vi "1_1_FFT and components.vi"() -> ()   [LabVIEW 2009]
doc: "This program calculates the magnitude spectrum, phase spectrum, real and imaginary spectrum of a sequence defined by the \"SIGNAL\" option menu."
uses:
  <vilib>/measure/matone.llb/Extract Single Tone Information 1 Chan.vi
  <vilib>/Analysis/2dsp.llb/Real FFT.vi
  <vilib>/Analysis/4window.llb/Hanning Window (DBL).vi
  <vilib>/Analysis/4window.llb/Hamming Window (DBL).vi
  <vilib>/Analysis/4window.llb/Triangle Window (DBL).vi
  <vilib>/Analysis/4window.llb/Kaiser-Bessel Window (DBL).vi
  <vilib>/Analysis/NI_AALBase.lvlib
  <vilib>/measure/NI_MAPro.lvlib
  <vilib>/Analysis/NI_AALPro.lvlib
panel:
  out "fft Phase":dbl[](array[numeric])=[nan, nan, nan, nan, nan, nan, nan, nan, nan, nan, nan, nan, nan, nan, nan, nan, nan, nan, nan, nan, nan, nan, nan, nan, nan, nan, nan, nan, nan, nan, nan, nan, nan, nan, nan, nan, nan, nan, nan, nan, nan, nan, nan, nan, nan, nan, nan, nan, nan, nan, nan, nan, nan, nan, nan, nan, nan, nan, nan, nan, nan, nan, nan, nan, nan, nan, nan, nan, nan, nan, nan, nan, nan, nan, nan, nan, nan, nan, nan, nan, nan, nan, nan, nan, nan, nan, nan, nan, nan, nan, nan, nan, nan, nan, nan, nan, nan, nan, nan, nan]
  out "fft Mag":dbl[](array[numeric])=[nan, nan, nan, nan, nan, nan, nan, nan, nan, nan, nan, nan, nan, nan, nan, nan, nan, nan, nan, nan, nan, nan, nan, nan, nan, nan, nan, nan, nan, nan, nan, nan, nan, nan, nan, nan, nan, nan, nan, nan, nan, nan, nan, nan, nan, nan, nan, nan, nan, nan, nan, nan, nan, nan, nan, nan, nan, nan, nan, nan, nan, nan, nan, nan, nan, nan, nan, nan, nan, nan, nan, nan, nan, nan, nan, nan, nan, nan, nan, nan, nan, nan, nan, nan, nan, nan, nan, nan, nan, nan, nan, nan, nan, nan, nan, nan, nan, nan, nan, nan]
  out "Freq res":dbl=10.0
  in  "Deg/Rad":enum16{"Rad", "Deg"}(ring)
  in  "Phase correction":bool
  out "FFT PHASE PLOT":cluster{dbl, "fundamental frequency":dbl, dbl[]}(graph)={-490.0, "fundamental frequency"=10.0, [0.0, 0.0, 0.0, 0.0, 0.15707963267948985, -0.0, -0.0, -0.0, -0.0, 0.0, 0.0, 0.0, 0.0, 0.0, 0.47123889803846863, -0.0, -0.0, -0.0, -0.0, -0.0, 0.0, 0.0, 0.0, 0.0, 0.7853981633974483, -0.0, -0.0, -0.0, -0.0, -0.0, 0.0, 0.0, 0.0, 0.0, 1.099557428756428, -0.0, -0.0, -0.0, -0.0, -0.0, 0.0, 0.0, 0.0, 0.0, 1.4137166941154071, -0.0, -0.0, -0.0, -0.0, 0.0, 0.0, 0.0, 0.0, 0.0, -1.4137166941154071, -0.0, -0.0, -0.0, -0.0, 0.0, 0.0, 0.0, 0.0, 0.0, -1.099557428756428, -0.0, -0.0, -0.0, -0.0, 0.0, 0.0, 0.0, 0.0, 0.0, -0.7853981633974483, -0.0, -0.0, -0.0, -0.0, 0.0, 0.0, 0.0, 0.0, 0.0, -0.47123889803846863, -0.0, -0.0, -0.0, -0.0, -0.0, 0.0, 0.0, 0.0, 0.0, -0.15707963267948985, -0.0, -0.0, -0.0, -0.0, 0.0]}
  out "FFT MAGNITUDE  PLOT":cluster{dbl, "fundamental frequency":dbl, dbl[]}(graph)={-490.0, "fundamental frequency"=10.0, [0.0, 0.0, 0.0, 0.0, 0.10124651257880031, 0.0, 0.0, 0.0, 0.0, 0.0, 0.0, 0.0, 0.0, 0.0, 0.11223262376343608, 0.0, 0.0, 0.0, 0.0, 0.0, 0.0, 0.0, 0.0, 0.0, 0.14142135623730956, 0.0, 0.0, 0.0, 0.0, 0.0, 0.0, 0.0, 0.0, 0.0, 0.22026892645852672, 0.0, 0.0, 0.0, 0.0, 0.0, 0.0, 0.0, 0.0, 0.0, 0.6392453221499662, 0.0, 0.0, 0.0, 0.0, 0.0, 0.0, 0.0, 0.0, 0.0, 0.6392453221499662, 0.0, 0.0, 0.0, 0.0, 0.0, 0.0, 0.0, 0.0, 0.0, 0.22026892645852672, 0.0, 0.0, 0.0, 0.0, 0.0, 0.0, 0.0, 0.0, 0.0, 0.14142135623730956, 0.0, 0.0, 0.0, 0.0, 0.0, 0.0, 0.0, 0.0, 0.0, 0.11223262376343608, 0.0, 0.0, 0.0, 0.0, 0.0, 0.0, 0.0, 0.0, 0.0, 0.10124651257880031, 0.0, 0.0, 0.0, 0.0, 0.0]}
  out "Imag arrray":dbl[](array[numeric])=[nan, nan, nan, nan, nan, nan, nan, nan, nan, nan, nan, nan, nan, nan, nan, nan, nan, nan, nan, nan, nan, nan, nan, nan, nan, nan, nan, nan, nan, nan, nan, nan, nan, nan, nan, nan, nan, nan, nan, nan, nan, nan, nan, nan, nan, nan, nan, nan, nan, nan, nan, nan, nan, nan, nan, nan, nan, nan, nan, nan, nan, nan, nan, nan, nan, nan, nan, nan, nan, nan, nan, nan, nan, nan, nan, nan, nan, nan, nan, nan, nan, nan, nan, nan, nan, nan, nan, nan, nan, nan, nan, nan, nan, nan, nan, nan, nan, nan, nan, nan]
  out "IMAGINARY  SPECTRUM":cluster{dbl, "fundamental frequency":dbl, dbl[]}(graph)={-490.0, "fundamental frequency"=10.0, [0.0, 0.0, 0.0, 0.0, 0.01583844403245365, -0.0, -0.0, -0.0, -0.0, 0.0, 0.0, 0.0, 0.0, 0.0, 0.050952544949442846, -0.0, -0.0, -0.0, -0.0, -0.0, 0.0, 0.0, 0.0, 0.0, 0.10000000000000003, -0.0, -0.0, -0.0, -0.0, -0.0, 0.0, 0.0, 0.0, 0.0, 0.19626105055051515, -0.0, -0.0, -0.0, -0.0, -0.0, 0.0, 0.0, 0.0, 0.0, 0.6313751514675043, -0.0, -0.0, -0.0, -0.0, 0.0, 0.0, 0.0, 0.0, 0.0, -0.6313751514675043, -0.0, -0.0, -0.0, -0.0, 0.0, 0.0, 0.0, 0.0, 0.0, -0.19626105055051515, -0.0, -0.0, -0.0, -0.0, 0.0, 0.0, 0.0, 0.0, 0.0, -0.10000000000000003, -0.0, -0.0, -0.0, -0.0, 0.0, 0.0, 0.0, 0.0, 0.0, -0.050952544949442846, -0.0, -0.0, -0.0, -0.0, -0.0, 0.0, 0.0, 0.0, 0.0, -0.01583844403245365, -0.0, -0.0, -0.0, -0.0, 0.0]}
  out "real arrray":dbl[](array[numeric])=[nan, nan, nan, nan, nan, nan, nan, nan, nan, nan, nan, nan, nan, nan, nan, nan, nan, nan, nan, nan, nan, nan, nan, nan, nan, nan, nan, nan, nan, nan, nan, nan, nan, nan, nan, nan, nan, nan, nan, nan, nan, nan, nan, nan, nan, nan, nan, nan, nan, nan, nan, nan, nan, nan, nan, nan, nan, nan, nan, nan, nan, nan, nan, nan, nan, nan, nan, nan, nan, nan, nan, nan, nan, nan, nan, nan, nan, nan, nan, nan, nan, nan, nan, nan, nan, nan, nan, nan, nan, nan, nan, nan, nan, nan, nan, nan, nan, nan, nan, nan]
  out "REAL SPECTRUM":cluster{dbl, "fundamental frequency":dbl, dbl[]}(graph)={-490.0, "fundamental frequency"=10.0, [0.0, 0.0, 0.0, 0.0, 0.10000000000000002, 0.0, 0.0, 0.0, 0.0, 0.0, 0.0, 0.0, 0.0, 0.0, 0.10000000000000002, 0.0, 0.0, 0.0, 0.0, 0.0, 0.0, 0.0, 0.0, 0.0, 0.10000000000000003, 0.0, 0.0, 0.0, 0.0, 0.0, 0.0, 0.0, 0.0, 0.0, 0.09999999999999995, 0.0, 0.0, 0.0, 0.0, 0.0, 0.0, 0.0, 0.0, 0.0, 0.09999999999999996, 0.0, 0.0, 0.0, 0.0, 0.0, 0.0, 0.0, 0.0, 0.0, 0.09999999999999996, 0.0, 0.0, 0.0, 0.0, 0.0, 0.0, 0.0, 0.0, 0.0, 0.09999999999999995, 0.0, 0.0, 0.0, 0.0, 0.0, 0.0, 0.0, 0.0, 0.0, 0.10000000000000003, 0.0, 0.0, 0.0, 0.0, 0.0, 0.0, 0.0, 0.0, 0.0, 0.10000000000000002, 0.0, 0.0, 0.0, 0.0, 0.0, 0.0, 0.0, 0.0, 0.0, 0.10000000000000002, 0.0, 0.0, 0.0, 0.0, 0.0]}
  in  "ARRAY DEFINED":dbl[](array[numeric])
  in  "Delta t":dbl=0.1 format="%0.2f"
  in  "Duty cycle (%)":dbl=50.0 format="%0.2f"
  in  "Width":i32=99
  in  "Start":dbl format="%0.2f"
  in  "End":dbl=1.0 format="%0.2f"
  in  "Reset phase":bool=TRUE
  in  "DELAY":dbl(knob) min=0.0 max=100.0 scale=0.0..100.0
  in  "AMPLITUDE":dbl=1.0 min=0.0 max=5.0 step=0.01 format="%#_6f"
  in  "PHASE IN":dbl(knob) scale=0.0..180.0
  in  "SIGNAL FREQUENCY":dbl(knob)=50.0 scale=0.0..10000.0 scale format="%#_6p"
  out "?":bool
  out "?":bool=TRUE
  in  "?":bool
  in  "Length":i32=100
  in  "Beta":dbl=5.0
  in  "Window":T1(ring)=enum."No window"
  out "?":bool
  out "?":bool
  out "DETECTED FREQUENCY":dbl=0.05 format="%.2p"
  out "# OF CYCLES":dbl=5.0
  out "?":string="SAMPLE"
  in  "?":bool
  out "TIME DOMAIN ORIGINAL SIGNAL":T2(graph)={0, "# OF SAMPLES"=1.0, "Sinc Pattern"=[1.0, 1.0, 1.0, 1.0, 1.0, 1.0, 1.0, 1.0, 1.0, 1.0, -1.0, -1.0, -1.0, -1.0, -1.0, -1.0, -1.0, -1.0, -1.0, -1.0, 1.0, 1.0, 1.0, 1.0, 1.0, 1.0, 1.0, 1.0, 1.0, 1.0, -1.0, -1.0, -1.0, -1.0, -1.0, -1.0, -1.0, -1.0, -1.0, -1.0, 1.0, 1.0, 1.0, 1.0, 1.0, 1.0, 1.0, 1.0, 1.0, 1.0, -1.0, -1.0, -1.0, -1.0, -1.0, -1.0, -1.0, -1.0, -1.0, -1.0, 1.0, 1.0, 1.0, 1.0, 1.0, 1.0, 1.0, 1.0, 1.0, 1.0, -1.0, -1.0, -1.0, -1.0, -1.0, -1.0, -1.0, -1.0, -1.0, -1.0, 1.0, 1.0, 1.0, 1.0, 1.0, 1.0, 1.0, 1.0, 1.0, 1.0, -1.0, -1.0, -1.0, -1.0, -1.0, -1.0, -1.0, -1.0, -1.0, -1.0]}
  in  "SAMPLING\nFREQUENCY (Hz)":dbl(slide)=1000.0 scale=0.0..20000.0 scale format="%#_6p"
  in  "# OF SAMPLES":dbl=100.0
  in  "SIGNAL":T3(ring)=enum."SQUARE"
  in  "stop":bool
  out "TIME DOMAIN WINDOWED SIGNAL":cluster{i32, dbl, "Sinc Pattern":dbl[]}[](graph)=[{0, 1.0, "Sinc Pattern"=[1.0, 1.0, 1.0, 1.0, 1.0, 1.0, 1.0, 1.0, 1.0, 1.0, -1.0, -1.0, -1.0, -1.0, -1.0, -1.0, -1.0, -1.0, -1.0, -1.0, 1.0, 1.0, 1.0, 1.0, 1.0, 1.0, 1.0, 1.0, 1.0, 1.0, -1.0, -1.0, -1.0, -1.0, -1.0, -1.0, -1.0, -1.0, -1.0, -1.0, 1.0, 1.0, 1.0, 1.0, 1.0, 1.0, 1.0, 1.0, 1.0, 1.0, -1.0, -1.0, -1.0, -1.0, -1.0, -1.0, -1.0, -1.0, -1.0, -1.0, 1.0, 1.0, 1.0, 1.0, 1.0, 1.0, 1.0, 1.0, 1.0, 1.0, -1.0, -1.0, -1.0, -1.0, -1.0, -1.0, -1.0, -1.0, -1.0, -1.0, 1.0, 1.0, 1.0, 1.0, 1.0, 1.0, 1.0, 1.0, 1.0, 1.0, -1.0, -1.0, -1.0, -1.0, -1.0, -1.0, -1.0, -1.0, -1.0, -1.0]}, {0, 1.0, "Sinc Pattern"=[1.0, 1.0, 1.0, 1.0, 1.0, 1.0, 1.0, 1.0, 1.0, 1.0, -1.0, -1.0, -1.0, -1.0, -1.0, -1.0, -1.0, -1.0, -1.0, -1.0, 1.0, 1.0, 1.0, 1.0, 1.0, 1.0, 1.0, 1.0, 1.0, 1.0, -1.0, -1.0, -1.0, -1.0, -1.0, -1.0, -1.0, -1.0, -1.0, -1.0, 1.0, 1.0, 1.0, 1.0, 1.0, 1.0, 1.0, 1.0, 1.0, 1.0, -1.0, -1.0, -1.0, -1.0, -1.0, -1.0, -1.0, -1.0, -1.0, -1.0, 1.0, 1.0, 1.0, 1.0, 1.0, 1.0, 1.0, 1.0, 1.0, 1.0, -1.0, -1.0, -1.0, -1.0, -1.0, -1.0, -1.0, -1.0, -1.0, -1.0, 1.0, 1.0, 1.0, 1.0, 1.0, 1.0, 1.0, 1.0, 1.0, 1.0, -1.0, -1.0, -1.0, -1.0, -1.0, -1.0, -1.0, -1.0, -1.0, -1.0]}]
  # "FFT and Components"
  # "SAMPLING INFO"
  # "Program developed by Indranil Sinharoy"
  # "ORIGINAL SIGNAL \nCHARACTERISTICS"
  # "RAMP"
  # "PULSE"
  # "SQUARE"
  # "SINC"
  # "View original\n     signal"
  # "View windowed\n        signal"
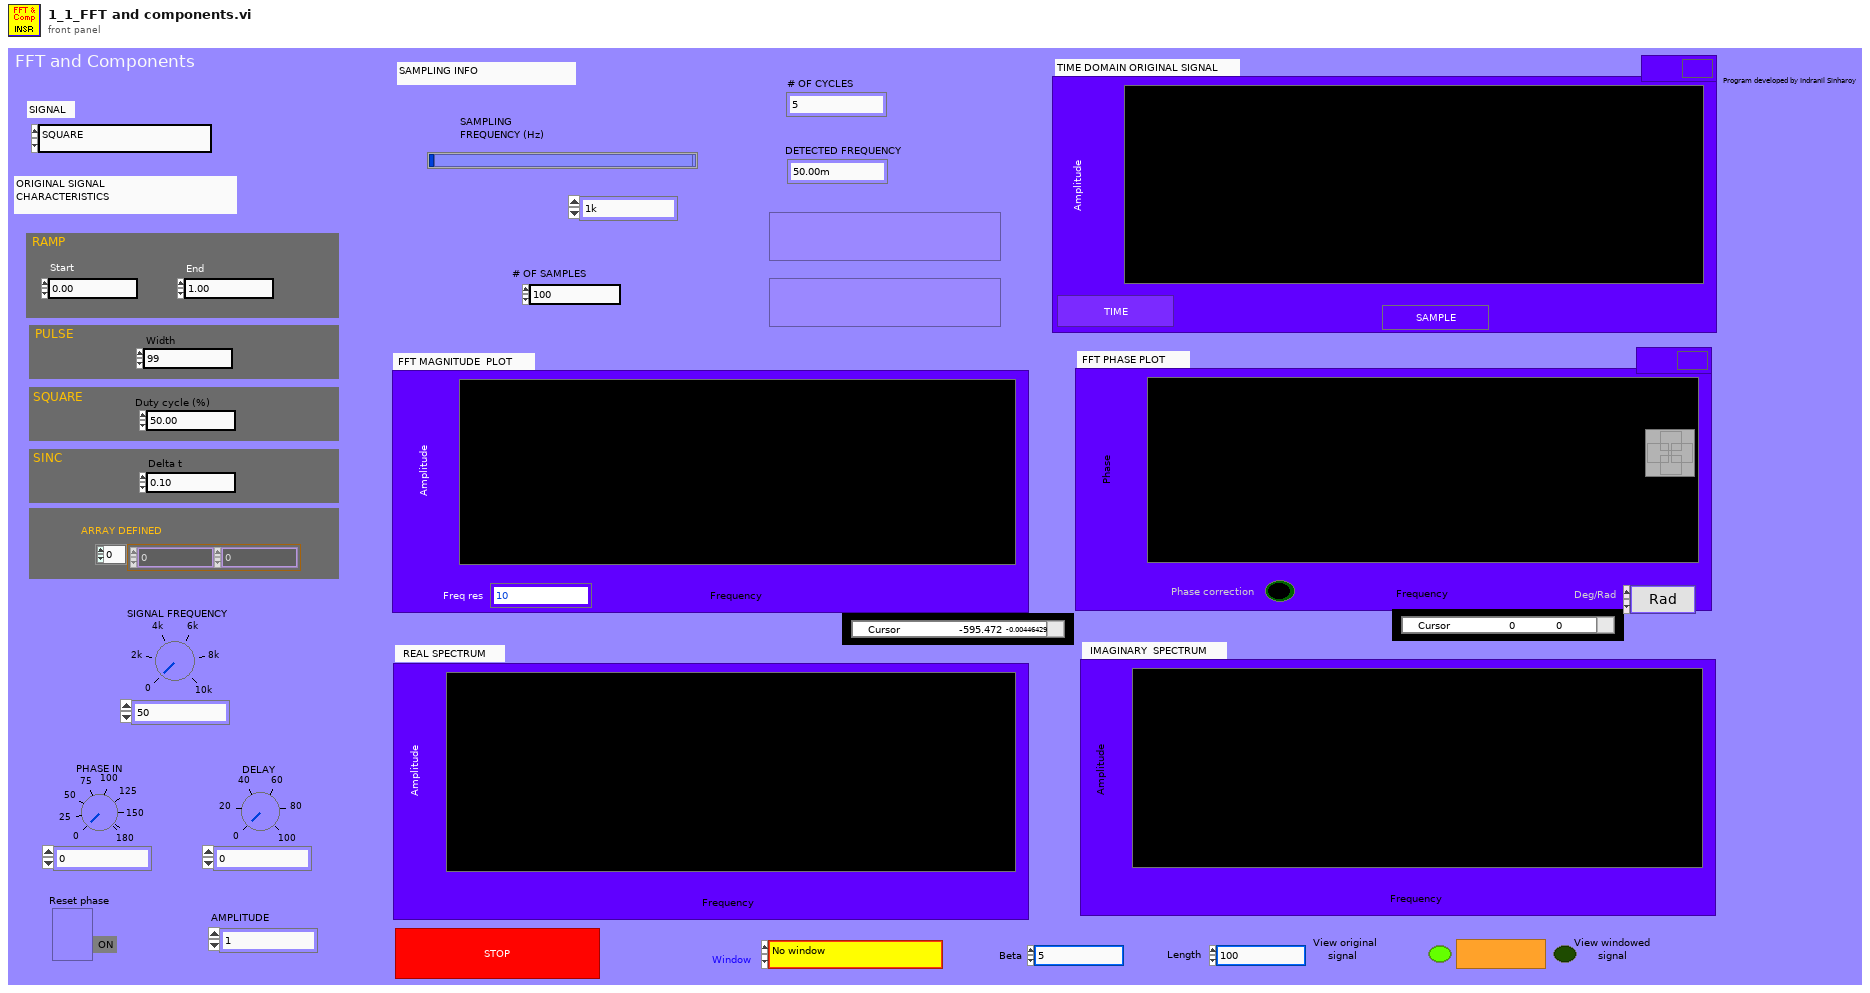
[diagram p1: front panel]
types:
  T1 = enum16{"Rectangular", "Hanning", "Hamming", "Triangular", "Kaiser-Bessel", "No window"}
  T2 = cluster{i32, "# OF SAMPLES":dbl, "Sinc Pattern":dbl[]}
  T3 = enum16{"SINE", "TRIANGULAR", "RAMP", "IMPULSE", "SINC ", "PULSE", "SQUARE", "ARRAY DEFINED"}
  T4 = cluster{dbl, "fundamental frequency":dbl, "reversed array":cdb[]}
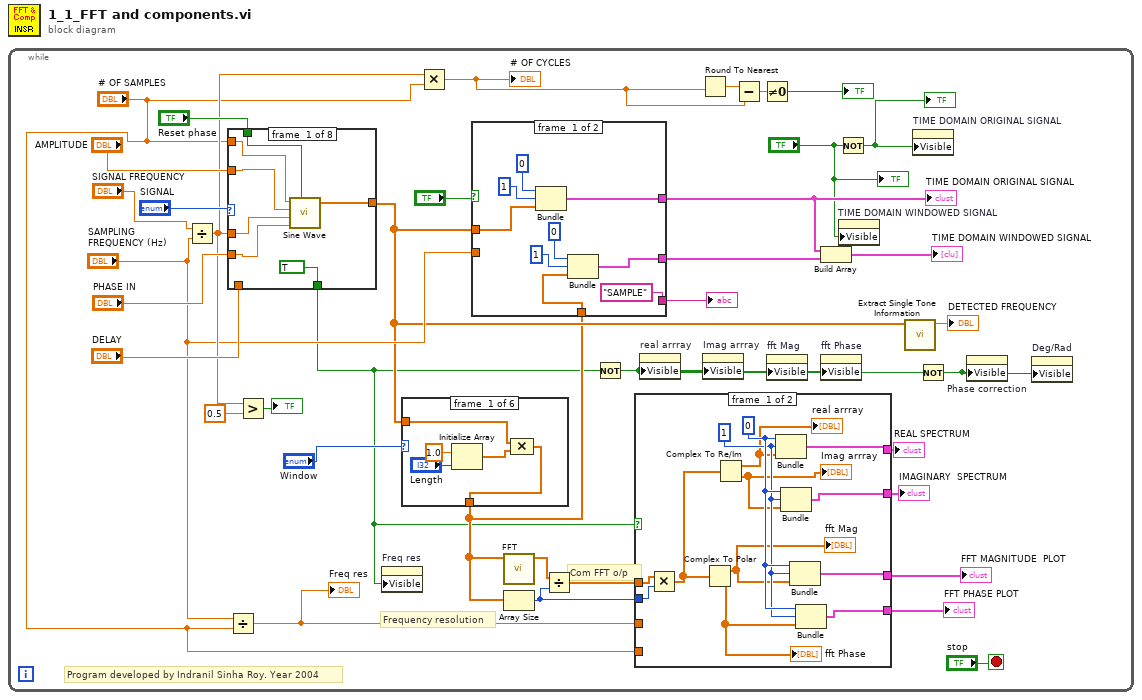
[diagram p0: block diagram]
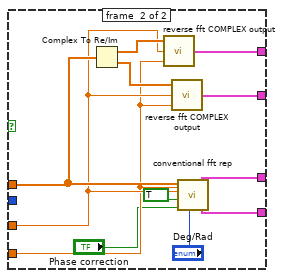
[diagram p2: hidden frame]
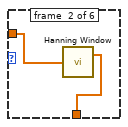
[diagram p3: hidden frame]
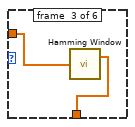
[diagram p4: hidden frame]
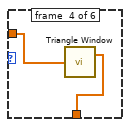
[diagram p5: hidden frame]
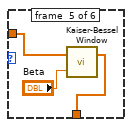
[diagram p6: hidden frame]
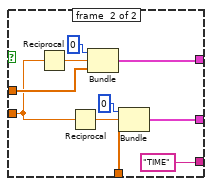
[diagram p8: hidden frame]
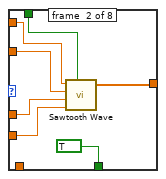
[diagram p9: hidden frame]
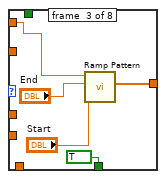
[diagram p10: hidden frame]
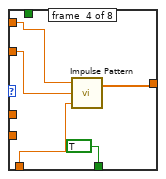
[diagram p11: hidden frame]
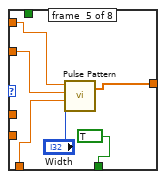
[diagram p12: hidden frame]
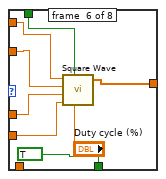
[diagram p13: hidden frame]
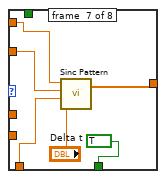
[diagram p14: hidden frame]
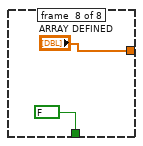
[diagram p15: hidden frame]
diagram:
  n1 = while {
    stop <- "stop" stop-if-true
    # "Program developed by Indranil Sinha Roy. Year 2004"
    # "Frequency resolution"
    # "Com FFT o/p"
    n2 = Divide(x="SIGNAL FREQUENCY", y="SAMPLING\nFREQUENCY (Hz)") -> (x/y=w27:dbl)
    n3 = case shown="\"ARRAY DEFINED\"" "SIGNAL" {
      tunnel: "Reset phase" -> [w104 w111 _ _ _ w135 _ _]
      tunnel: "AMPLITUDE" -> [w102 w109 _ w120 w126 w133 w140 _]
      tunnel: "# OF SAMPLES" -> [w103 w110 w115 w121 w127 w134 w141 _]
      tunnel: w27 -> [w101 w108 _ _ _ w132 _ _]
      tunnel: "PHASE IN" -> [w100 w107 _ _ _ w131 _ _]
      tunnel: "DELAY" -> [_ _ _ w119 w125 _ w139 _]
      tunnel: [w99 w106 w116 w118 w124 w130 w138 "ARRAY DEFINED"] -> w12
      tunnel: [TRUE TRUE TRUE TRUE TRUE TRUE TRUE FALSE] -> w2
      frame #0 {
        n4 = call <vilib>:"Sine Wave.vi"("samples"=w103, "amplitude"=w102, "frequency"=w101, "phase in"=w100, "reset phase"=w104) -> ("sine wave"=w99:dbl[])  [unwired: 2 out]
      }
      frame #1 {
        n5 = call <vilib>:"Sawtooth Wave.vi"("samples"=w110, "amplitude"=w109, "frequency"=w108, "phase in"=w107, "reset phase"=w111) -> ("sawtooth wave"=w106:dbl[])  [unwired: 2 out]
      }
      frame #2 {
        n6 = call <vilib>:"Ramp Pattern.vi"("start"="Start", "end"="End", "samples"=w115) -> ("Ramp Pattern"=w116:dbl[])  [unwired: 7 in, 1 out]
      }
      frame #3 {
        n7 = call <vilib>:"Impulse Pattern.vi"("delay"=w119, "amplitude"=w120, "samples"=w121) -> ("Impulse Pattern"=w118:dbl[])  [unwired: 1 out]
      }
      frame #4 {
        n8 = call <vilib>:"Pulse Pattern.vi"("width"="Width", "delay"=w125, "amplitude"=w126, "samples"=w127) -> ("Pulse Pattern"=w124:dbl[])  [unwired: 1 out]
      }
      frame #5 {
        n9 = call <vilib>:"Square Wave.vi"("samples"=w134, "reset phase"=w135, "amplitude"=w133, "frequency"=w132, "duty cycle (%)"="Duty cycle (%)", "phase in"=w131) -> ("square wave"=w130:dbl[])  [unwired: 2 out]
      }
      frame #6 {
        n10 = call <vilib>:"Sinc Pattern.vi"("delta t"="Delta t", "delay"=w139, "amplitude"=w140, "samples"=w141) -> ("Sinc Pattern"=w138:dbl[])  [unwired: 1 out]
      }
      frame #7 {
      }
    }
    n11 = Divide(x="SAMPLING\nFREQUENCY (Hz)", y="# OF SAMPLES") -> (x/y=w3:dbl)
    "Freq res" <- w3
    n12 = Greater?(x=w27, y=0.5) -> (0:→"?":bool)
    n13 = property on="Freq res" class="DigNum (strict)"("Visible"=w2) -> ()  [unwired: 2 in, 2 out]
    n14 = case shown="\"Rectangular\", Default" "Window" {
      tunnel: w12 -> [w66 w70 w72 w74 w77 w78]
      tunnel: [w65 w69 w71 w73 w76 w78] -> w11
      frame #0 {
        n15 = Initialize Array(1.0 ("element"), "Length") -> (w67:dbl[])
        n16 = Compound Arithmetic op=MULTIPLY(w66, w67) -> (w65:dbl[])
      }
      frame #1 {
        n17 = call-poly <vilib>:"Hanning Window.vi"("X"=w70) -> ("Windowed X"=w69:dbl[])  [unwired: 1 out]
      }
      frame #2 {
        n18 = call-poly <vilib>:"Hamming Window.vi"("X"=w72) -> ("Windowed X"=w71:dbl[])  [unwired: 1 out]
      }
      frame #3 {
        n19 = call-poly <vilib>:"Triangle Window.vi"("X"=w74) -> ("Windowed X"=w73:dbl[])  [unwired: 1 out]
      }
      frame #4 {
        n20 = call-poly <vilib>:"Kaiser-Bessel Window.vi"("beta"="Beta", "X"=w77) -> ("Windowed X"=w76:dbl[])  [unwired: 1 out]
      }
      frame #5 {
      }
    }
    n21 = Multiply(x=w27, y="# OF SAMPLES") -> (x*y=w24:dbl)
    "# OF CYCLES" <- w24
    n22 = case shown="False" "?" {
      tunnel: w12 -> [w86 w96]
      tunnel: [w84 w94] -> w9
      tunnel: "SAMPLING\nFREQUENCY (Hz)" -> [_ w89]
      tunnel: ["SAMPLE" "TIME"] -> w29
      tunnel: w11 -> [w80 w90]
      tunnel: [w79 w88] -> w10
      frame #0 {
        n23 = Bundle(0, 1, "ARRAY DEFINED"=w86) -> (w84:cluster{i32, i32, "ARRAY DEFINED":dbl[]})  [unwired: 1 in]
        n24 = Bundle(0, 1, "ARRAY DEFINED"=w80) -> (w79:cluster{i32, i32, "ARRAY DEFINED":dbl[]})  [unwired: 1 in]
      }
      frame #1 {
        n25 = Reciprocal(x=w89) -> (1/x=w97:dbl)
        n26 = Reciprocal(x=w89) -> (1/x=w91:dbl)
        n27 = Bundle(0, w97, "ARRAY DEFINED"=w96) -> (w94:cluster{i32, dbl, "ARRAY DEFINED":dbl[]})  [unwired: 1 in]
        n28 = Bundle(0, w91, "ARRAY DEFINED"=w90) -> (w88:cluster{i32, dbl, "ARRAY DEFINED":dbl[]})  [unwired: 1 in]
      }
    }
    "TIME DOMAIN ORIGINAL SIGNAL" <- w9
    "?" <- w29
    n29 = call-poly <vilib>:"FFT.vi"("X"=w11) -> ("FFT {X}"=w18:cdb[])  [unwired: 9 in, 1 out]
    n30 = Array Size(array=w11) -> (size(s)=w5:i32)
    n31 = Divide(x=w18, y=w5) -> (x/y=w17:cdb[])
    n32 = Not(x=w2) -> (.not. x?=w4:bool)
    n33 = case shown="False" w2 {
      tunnel: [w47 w63] -> w20
      tunnel: [w46 w62] -> w19
      tunnel: w17 -> [w44 w61]
      tunnel: [w49 w59] -> w16
      tunnel: w3 -> [_ w57]
      tunnel: "# OF SAMPLES" -> [_ w56]
      tunnel: [w48 w55] -> w14
      tunnel: w5 -> [w43 _]
      frame #0 {
        w50 = 1
        w51 = 0
        n34 = Multiply(x=w44, y=w43) -> (x*y=w45:cdb[])
        n35 = Complex To Polar(r * e^(i*theta)=w45) -> (r=w40:dbl[], theta=w41:dbl[])
        "fft Phase" <- w41
        "fft Mag" <- w40
        n36 = Complex To Re/Im(x + iy=w45) -> (x=w42:dbl[], y=w39:dbl[])
        "real arrray" <- w42
        "Imag arrray" <- w39
        n37 = Bundle(w51, w50, w42) -> (w49:cluster{i32, i32, dbl[]})  [unwired: 1 in]
        n38 = Bundle(w51, w50, w39) -> (w48:cluster{i32, i32, dbl[]})  [unwired: 1 in]
        n39 = Bundle(w51, w50, w40) -> (w47:cluster{i32, i32, dbl[]})  [unwired: 1 in]
        n40 = Bundle(w51, w50, w41) -> (w46:cluster{i32, i32, dbl[]})  [unwired: 1 in]
      }
      frame #1 {
        n41 = Complex To Re/Im(x + iy=w61) -> (x=w60:dbl[], y=w58:dbl[])
        n42 = call "reverse fft COMPLEX output.vi"("samples"=w56, "fundamental frequency"=w57, "fft output"=w60) -> ("Reversed FFT COMPLEX O/P"=w59:T4)
        n43 = call "reverse fft COMPLEX output.vi"("samples"=w56, "fundamental frequency"=w57, "fft output"=w58) -> ("Reversed FFT COMPLEX O/P"=w55:T4)
        n44 = call "conventional fft rep.vi"("Deg/Rad"="Deg/Rad", "samples"=w56, "Phase correction"="Phase correction", "Phase Unwrap"=TRUE, "fundamental frequency"=w57, "fft output"=w61) -> ("Conventional FFT phase"=w62:cluster{dbl, "fundamental frequency":dbl, dbl[]}, "Conventional FFT mag"=w63:cluster{dbl, "fundamental frequency":dbl, dbl[]})
      }
    }
    "FFT MAGNITUDE  PLOT" <- w20
    "FFT PHASE PLOT" <- w19
    "REAL SPECTRUM" <- w16
    "IMAGINARY  SPECTRUM" <- w14
    n45 = property on="real arrray" class="Arr (strict)"("Visible"=w4) -> ()  [unwired: 2 in, 2 out]
    n46 = Round To Nearest(number=w24) -> (nearest integer value=w25:dbl)
    n47 = property on="Imag arrray" class="Arr (strict)"("Visible"=w4) -> ()  [unwired: 2 in, 2 out]
    n48 = Subtract(x=w25, y=w24) -> (x-y=w23:dbl)
    n49 = Not Equal To 0?(x=w23) -> (x != 0?=→"?":bool)
    n50 = property on="fft Mag" class="Arr (strict)"("Visible"=w4) -> ()  [unwired: 2 in, 2 out]
    n51 = Build Array(w9, w10) -> (→"TIME DOMAIN WINDOWED SIGNAL":cluster{i32, dbl, "ARRAY DEFINED":dbl[]}[])
    n52 = property on="fft Phase" class="Arr (strict)"("Visible"=w4) -> ()  [unwired: 2 in, 2 out]
    n53 = Not(x="?") -> (.not. x?=w6:bool)
    "?" <- w6
    n54 = property on="TIME DOMAIN WINDOWED SIGNAL" class="WFGraph (strict)"("Visible"="?") -> ()  [unwired: 2 in, 2 out]
    n55 = call-poly <vilib>:"Extract Single Tone Information.vi"("time signal in"=w12) -> ("detected frequency"=→"DETECTED FREQUENCY":dbl)  [unwired: 5 in, 5 out]
    n56 = property on="TIME DOMAIN ORIGINAL SIGNAL" class="WFGraph (strict)"("Visible"=w6) -> ()  [unwired: 2 in, 2 out]
    n57 = Not(x=w4) -> (.not. x?=w1:bool)
    n58 = property on="Phase correction" class="Bool (strict)"("Visible"=w1) -> ()  [unwired: 2 in, 2 out]
    n59 = property on="Deg/Rad" class="Enum (strict)"("Visible"=w1) -> ()  [unwired: 2 in, 2 out]
    "?" <- "?"
  }
